vi "Simulate Keysight 34401a TCP.vi"() -> ()   [LabVIEW 2021]
uses:
  <vilib>/Utility/error.llb/Error Cluster From Error Code.vi
  <vilib>/Utility/config.llb/Read Key (String).vi
  <vilib>/ErrorRing/Error Ring.xnode
  <vilib>/Utility/config.llb/NI_LVConfig.lvlib
panel:
  out "error out":errorcluster
  in  "stop":bool
  in  "timeout ms (wait forever: -1)":i32=1000
  in  "port":u16=50000
  in  "error in":errorcluster
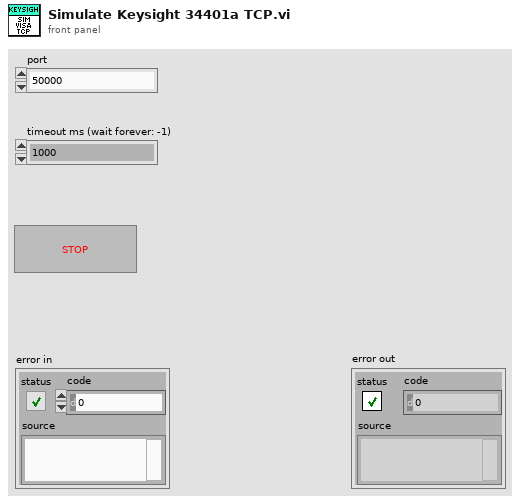
[diagram p1: front panel]
types:
  T1 = typedef "NI_LVConfig.lvlib/Config Data RefNum.ctl" = refnum<k1>
  T2 = enum16{"Standard", "Buffered", "CRLF", "Immediate"}
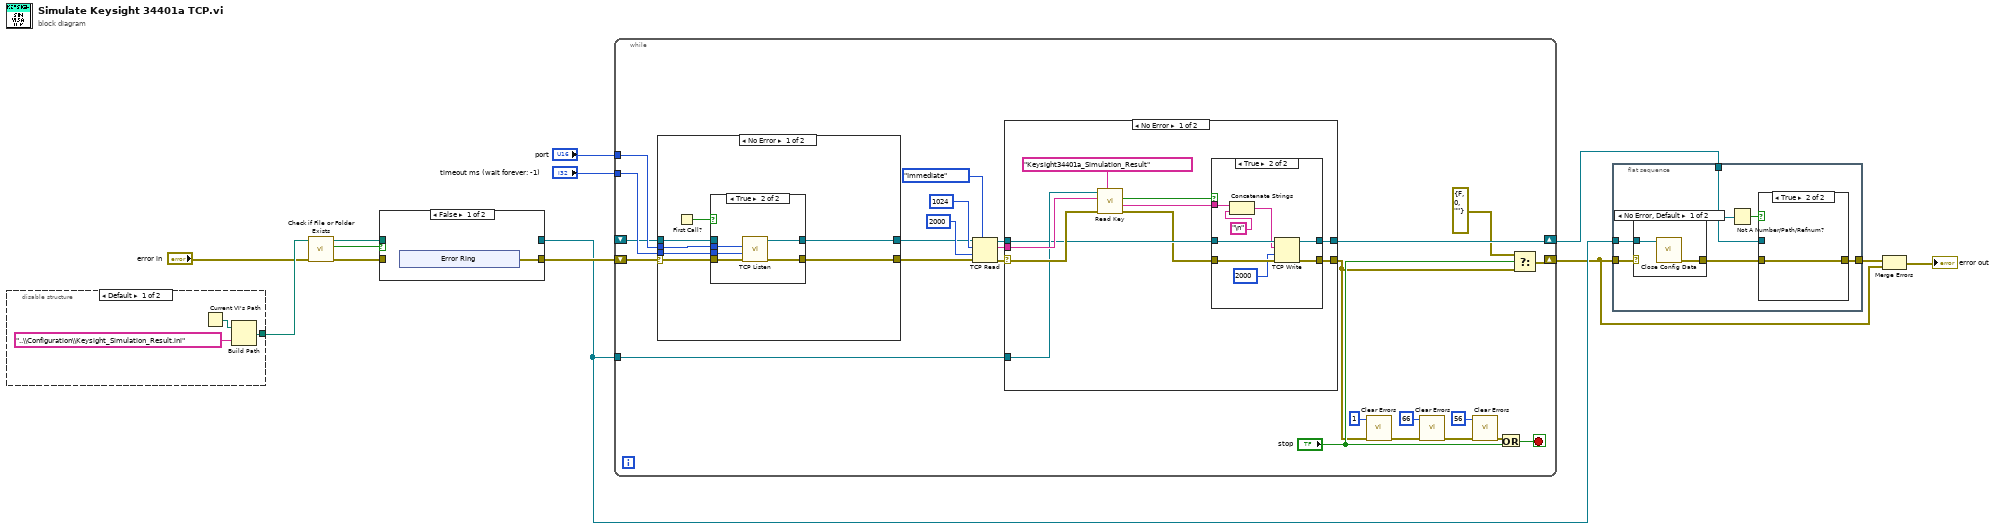
[diagram p0: block diagram]
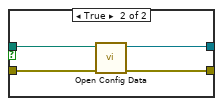
[diagram p2: hidden frame]
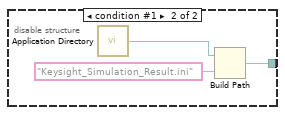
[diagram p3: hidden frame]
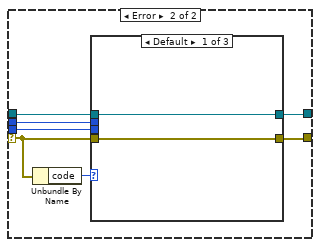
[diagram p7: hidden frame]
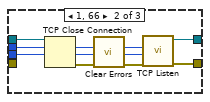
[diagram p8: hidden frame]
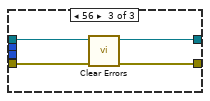
[diagram p9: hidden frame]
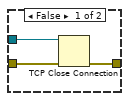
[diagram p11: hidden frame]
diagram:
  n1 = disable-structure shown="Default" {
    disable-tunnel: [w14 w19] -> w5
    frame condition #0 (active) {
      n2 = Current VI's Path() -> (path=w16:path)
      n3 = Build Path(base path=w16, name or relative path="..\\Configuration\\Keysight_Simulation_Result.ini" ("write buffer")) -> (appended path=w14:path)
    }
    frame condition #1 {
      n4 = call <vilib>:"Application Directory.vi"() -> ("Application Directory"=w17:path)
      n5 = Build Path(base path=w17, name or relative path="Keysight_Simulation_Result.ini" ("write buffer")) -> (appended path=w19:path)
    }
  }
  n6 = call <vilib>:"Check if File or Folder Exists.vi"("error in (no error)"="error in", "path"=w5) -> ("error out"=w3:errorcluster, "file or folder exists?"=w2:bool, "dup path"=w1:path)  [unwired: 7 in]
  n7 = case shown="False" w2 {
    tunnel: [w20 w29] -> w13
    tunnel: [_ w28] -> w12
    tunnel: w3 -> [_ w27]
    tunnel: w1 -> [_ w26]
    frame False {
      n8 = xnode "Error Ring"() -> ("error out"=w20:errorcluster)
    }
    frame True {
      n9 = call <vilib>:"Open Config Data.vi"("error in (no error)"=w27, "configuration file path"=w26) -> ("error out"=w29:errorcluster, "refnum"=w28:T1)  [unwired: 7 in, 1 out]
    }
  }
  n10 = while {
    tunnel: w12 -> [w49]
    tunnel: "port" -> [w42]
    tunnel: "timeout ms (wait forever: -1)" -> [w41]
    shift-right: [w30] -> w9
    shift-left: w13 -> [w43]
    shift-right: [w45] -> w8
    shift-left: _ -> [w36]
    stop <- w47 stop-if-true
    n11 = case shown="No Error" w43 {
      selector: w43 -> [w81 w95]
      tunnel: [w83 w94] -> w46
      tunnel: [w82 w96] -> w44
      tunnel: w42 -> [w80 w93]
      tunnel: w41 -> [w79 w92]
      tunnel: w36 -> [w77 w91]
      frame No Error {
        n12 = First Call?() -> (First Call?: T/F=w78:bool)
        n13 = case shown="True" w78 {
          tunnel: [w84 w90] -> w83
          tunnel: [w85 w89] -> w82
          tunnel: w81 -> [w85 w88]
          tunnel: w80 -> [_ w87]
          tunnel: w79 -> [_ w86]
          tunnel: w77 -> [w84 _]
          frame False {
          }
          frame True {
            n14 = call <vilib>:"TCP Listen.vi"("error in (no error)"=w88, "timeout ms (wait forever: -1)"=w86, "port"=w87) -> ("error out"=w89:errorcluster, "connection ID"=w90:refnum<k5>)  [unwired: 4 in, 3 out]
          }
        }
      }
      frame Error {
        n15 = Unbundle By Name(w95) -> ("code"=w97:i32)
        n16 = case shown="Default" w97 {
          tunnel: [w99 w106 w107] -> w96
          tunnel: w95 -> [w99 _ w109]
          tunnel: [w98 w105 w108] -> w94
          tunnel: w93 -> [_ w104 _]
          tunnel: w92 -> [_ w103 _]
          tunnel: w91 -> [w98 w101 w108]
          frame Default {
          }
          frame 1, 66 {
            n17 = TCP Close Connection(connection ID=w101) -> (error out=w102:errorcluster)  [unwired: 2 in, 1 out]
            n18 = call <vilib>:"Clear Errors.vi"("error in (no error)"=w102) -> ("error out"=w100:errorcluster)  [unwired: 5 in, 1 out]
            n19 = call <vilib>:"TCP Listen.vi"("error in (no error)"=w100, "timeout ms (wait forever: -1)"=w103, "port"=w104) -> ("error out"=w106:errorcluster, "connection ID"=w105:refnum<k5>)  [unwired: 4 in, 3 out]
          }
          frame 56 {
            n20 = call <vilib>:"Clear Errors.vi"("error in (no error)"=w109) -> ("error out"=w107:errorcluster)  [unwired: 5 in, 1 out]
          }
        }
      }
    }
    n21 = TCP Read(connection ID=w46, bytes to read=1024, error in (no error)=w44, 7:T2."Immediate" ("mode (standard)"), 9:2000 ("timeout ms (25000)")) -> (connection ID out=w48:refnum<k5>, data out=w50:string, error out=w51:errorcluster)
    n22 = case shown="No Error" w51 {
      selector: w51 -> [w64 w75]
      tunnel: w50 -> [w63 _]
      tunnel: w49 -> [w62 _]
      tunnel: w48 -> [w61 w76]
      tunnel: [w60 w75] -> w32
      tunnel: [w59 w76] -> w45
      frame No Error {
        n23 = call-poly <vilib>:"Read Key.vi"("section"="Keysight34401a_Simulation_Result", "error in (no error)"=w64, "key"=w63, "refnum"=w62) -> ("error out"=w57:errorcluster, "value"=w56:string, "found?"=w55:bool)  [unwired: 4 in, 1 out]
        n24 = case shown="True" w55 {
          tunnel: w57 -> [w66 w74]
          tunnel: [w66 w73] -> w60
          tunnel: w61 -> [w65 w72]
          tunnel: w56 -> [_ w70]
          tunnel: [w65 w69] -> w59
          frame False {
          }
          frame True {
            n25 = Concatenate Strings(w70, "\n") -> (w68:string)
            n26 = TCP Write(connection ID=w72, data in=w68, error in (no error)=w74, 9:2000 ("timeout ms (25000)")) -> (connection ID out=w69:refnum<k5>, error out=w73:errorcluster)  [unwired: 1 out]
          }
        }
      }
      frame Error {
      }
    }
    n27 = call <vilib>:"Clear Errors.vi"("error in (no error)"=w32, "specific error code to clear (0: all)"=1) -> ("error out"=w35:errorcluster)  [unwired: 4 in, 1 out]
    n28 = call <vilib>:"Clear Errors.vi"("error in (no error)"=w35, "specific error code to clear (0: all)"=66) -> ("error out"=w38:errorcluster)  [unwired: 4 in, 1 out]
    n29 = call <vilib>:"Clear Errors.vi"("error in (no error)"=w38, "specific error code to clear (0: all)"=56) -> ("error out"=w40:errorcluster)  [unwired: 4 in, 1 out]
    n30 = Or(x=w40, y="stop") -> (x .or. y?=w47:bool)
    n31 = Select(t=errorcluster {"status"=FALSE, "code"=0, "source"=""}, s="stop", f=w32) -> (s? t:f=w30:errorcluster)
  }
  n32 = flat-sequence {
    tunnel: w12 -> [w115]
    tunnel: [w113] -> w11
    tunnel: w8 -> [w112]
    tunnel: w9 -> [w110]
    frame #0 {
      n33 = case shown="No Error, Default" w110 {
        tunnel: w115 -> [w117 _]
        tunnel: [w116 _] -> w114
        frame No Error {
          n34 = call <vilib>:"Close Config Data.vi"("refnum"=w117) -> ("error out"=w116:errorcluster)  [unwired: 9 in, 1 out]
        }
        frame Error {
        }
      }
      n35 = Not A Number/Path/Refnum?(number/path/refnum=w112) -> (NaN/Path/Refnum?=w111:bool)
      n36 = case shown="True" w111 {
        tunnel: w114 -> [w120 w121]
        tunnel: [w119 w121] -> w113
        tunnel: w112 -> [w118 _]
        frame False {
          n37 = TCP Close Connection(connection ID=w118, error in (no error)=w120) -> (error out=w119:errorcluster)  [unwired: 1 in, 1 out]
        }
        frame True {
        }
      }
    }
  }
  n38 = Merge Errors(w11, w9) -> (→"error out":errorcluster)
